vi "Get Group Config Variables.vi"(8 "error in (no error)":errorcluster, 10 "Error":string, 11 "LabVIEW Web Service Request":refnum<class "Web Request.lvclass">) -> (0 "error out":errorcluster, 3 "LabVIEW Web Service Request out":refnum<class "Web Request.lvclass">)   [LabVIEW 2018]
doc: "This VI sets all of the ESP variables for a single contact so it can be output from an ESP script."
uses:
  <vilib>/wsapi/Web Request.lvclass
  subvis/Group Properties.ctl
  CAEN globals.vi
  <vilib>/wsapi/class/subVIs/Set Many String ESP Variables.vi
panel:
  in  "Group Prop":T1 caption="Property"
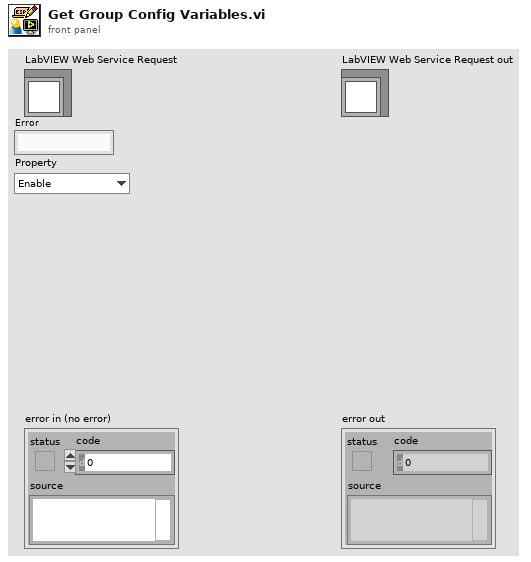
[diagram p1: front panel]
types:
  T1 = typedef "Group Properties.ctl" = enum16{"Enable", "Vset", "Imax", "Vswmax", "Trip Time"}
  T2 = typedef "channel.ctl" = cluster{" Card.Channel":dbl, "Crate":i32}
  T3 = cluster{"Group Name":string, "Channels in Group":T2[]}[]
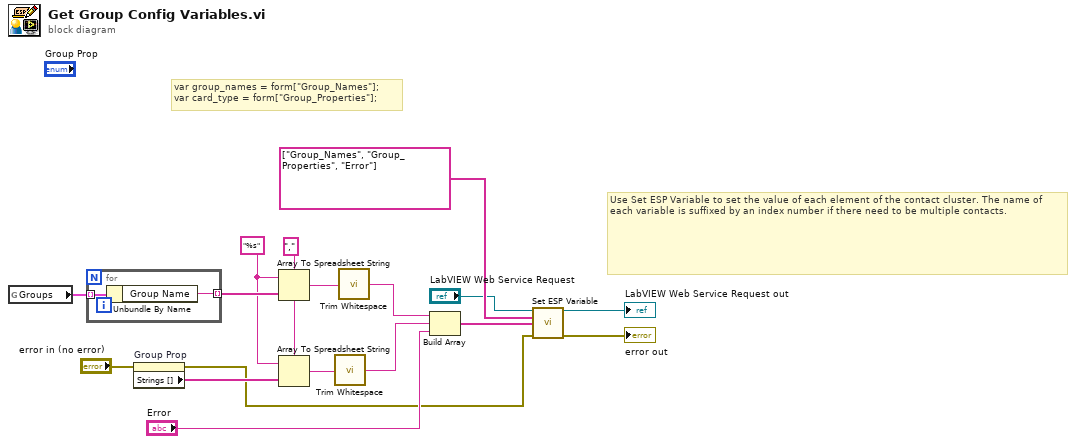
[diagram p0: block diagram]
diagram:
  w9 = "%s" ("delimiter (Tab)")
  w10 = "," ("delimiter (Tab)")
  # "var group_names = form[\"Group_Names\"];\nvar card_type = form[\"Group_Properties\"];"
  # "Use Set ESP Variable to set the value of each element of the contact cluster. The name of each variable is suffixed by an index number if there need to be multiple contacts."
  n1 = global read "CAEN globals.vi" "Groups"() -> (w12:T3)
  n2 = for {
    tunnel: w12 -> [w19] mode=indexing
    tunnel: [w18] -> w11 mode=indexing
    n3 = Unbundle By Name(w19) -> ("Group Name"=w18:string)
  }
  n4 = property on="Group Prop" class="Enum (strict)"(error in="error in (no error)") -> (error out=w1:errorcluster, "Strings []"=w2:string[])  [unwired: 1 in, 1 out]
  n5 = Array To Spreadsheet String(delimiter (Tab)=w10, array=w11, 3:w9) -> (spreadsheet string=w7:string)
  n6 = Array To Spreadsheet String(delimiter (Tab)=w10, array=w2, 3:w9) -> (spreadsheet string=w5:string)
  n7 = call <vilib>:"Trim Whitespace.vi"("string"=w5) -> ("trimmed string"=w4:string)  [unwired: 1 in]
  n8 = call <vilib>:"Trim Whitespace.vi"("string"=w7) -> ("trimmed string"=w6:string)  [unwired: 1 in]
  n9 = Build Array(w6, w4, "Error") -> (w16:string[])
  n10 = call-poly <vilib>:"Set ESP Variable.vi"("LabVIEW Web Service Request"="LabVIEW Web Service Request", "keys"=string[] ["Group_Names", "Group_Properties", "Error"] ("appended array"), "values"=w16, "error in (no error)"=w1) -> ("LabVIEW Web Service Request out"=→"LabVIEW Web Service Request out":refnum<class "Web Request.lvclass">, "error out"=→"error out":errorcluster)  [unwired: 10 in]
